vi "Write inner terminals.vi"(5 "inner terminals":refnum<class "Terminal.lvclass">[](array[class]), 9 "Tunnel in":refnum<class "Tunnel.lvclass">) -> (3 "Tunnel out":refnum<class "Tunnel.lvclass">)   [LabVIEW 2014, in "Raspberry Pi Compatible Compiler for LabVIEW.lvlib" / "Tunnel.lvclass"]
uses:
  Tunnel.lvclass
  Terminal/Terminal.lvclass
  Tunnel.lvclass/Tunnel.ctl
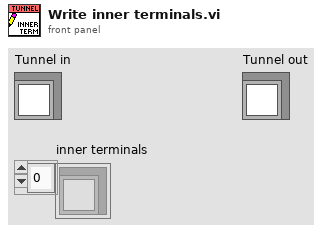
[diagram p1: front panel]
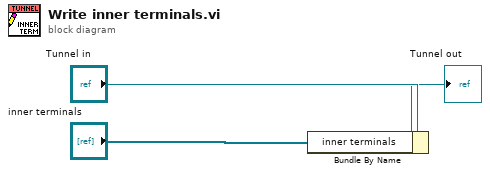
[diagram p0: block diagram]
diagram:
  n1 = Bundle By Name(cluster="Tunnel in", "inner terminals"="inner terminals") -> (→"Tunnel out":refnum<class "Tunnel.lvclass">)
